vi "digir detector.vi"() -> ()   [LabVIEW 2018]
panel:
  out "Array":dbl[](array[numeric])
  out "Waveform Graph":dbl[](graph)
  out "substring":string
  out "0<=data<=9":bool
  in  "input string":string
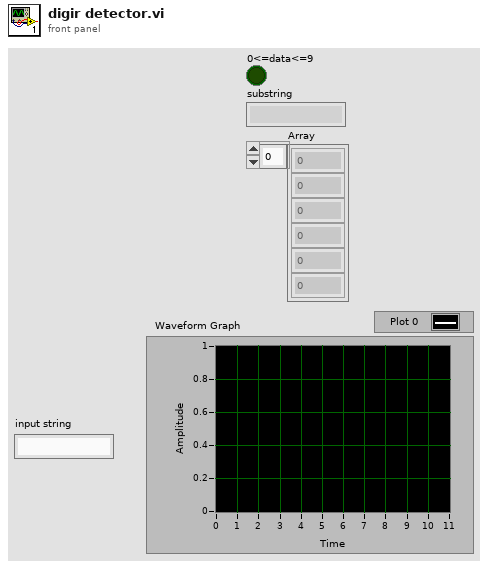
[diagram p1: front panel]
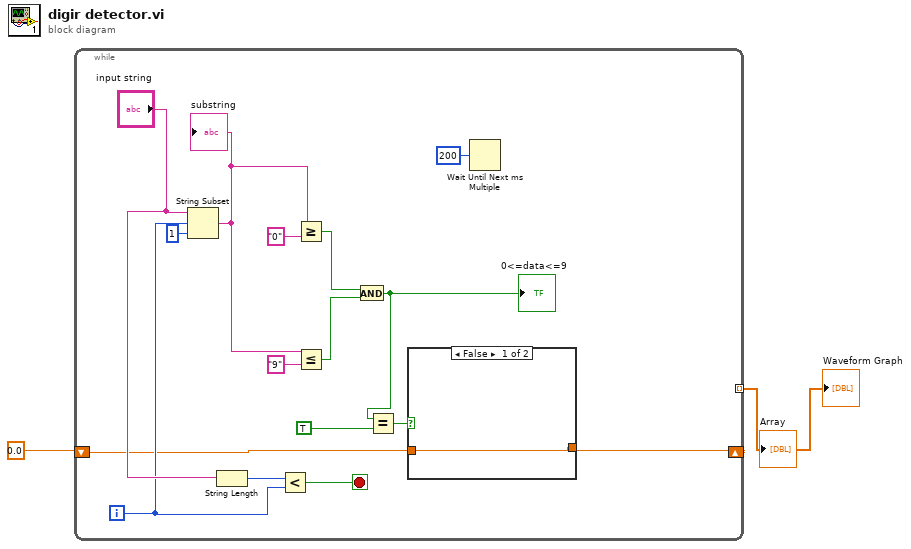
[diagram p0: block diagram]
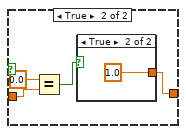
[diagram p2: hidden frame]
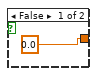
[diagram p3: hidden frame]
diagram:
  n1 = while {
    shift-right: [w3] -> _
    shift-left: 0.0 -> [w5]
    tunnel: [w3] -> w1 mode=indexing
    i -> [w11]
    stop <- w9 stop-if-true
    n2 = String Subset(string="input string", offset (0)=w11, length (rest)=1 ("length (rest)")) -> (substring=w13:string)
    "substring" <- w13
    n3 = String Length(string="input string") -> (length=w10:i32)
    n4 = Less?(x=w10, y=w11) -> (x < y?=w9:bool)
    n5 = Greater Or Equal?(x=w13, y="0") -> (x >= y?=w17:bool)
    n6 = Less Or Equal?(x=w13, y="9") -> (x <= y?=w16:bool)
    n7 = And(x=w17, y=w16) -> (x .and. y?=w8:bool)
    "0<=data<=9" <- w8
    n8 = Equal?(x=w8, y=TRUE) -> (x = y?=w6:bool)
    n9 = case shown="False" w6 {
      tunnel: w5 -> [w19 w23]
      tunnel: [w19 w20] -> w3
      frame False {
      }
      frame True {
        n10 = Equal?(x=0.0, y=w23) -> (x = y?=w21:bool)
        n11 = case shown="True" w21 {
          tunnel: [0.0 1.0] -> w20
          frame False {
          }
          frame True {
          }
        }
      }
    }
    n12 = Wait Until Next ms Multiple(millisecond multiple=u32 200) -> ()  [unwired: 1 out]
  }
  "Waveform Graph" <- w1
  "Array" <- w1
